vi "FPGA_GetRef.vi"() -> (0 "error out":errorcluster, 2 "FPGA_Ref":refnum<k20>)   [LabVIEW 2009]
uses:
  <vilib>/rvi/interface/nirviOpenFPGA/nirviOpenFPGA.xnode
  FPGA Bitfiles/scmproject.lvproj_FPGA Target_RobotFPGA.vi.lvbitx
  RobotFPGA.vi
  <vilib>/FPGAPlugInAG/cRIO-9074/nirviIntfOpen_cRIO-9074.vi
  <vilib>/userdefined/High Color/nirio_resource_hc.ctl
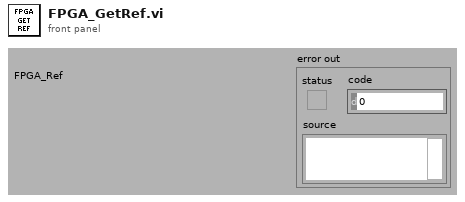
[diagram p1: front panel]
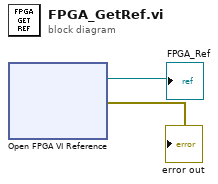
[diagram p0: block diagram]
diagram:
  n1 = xnode "Open FPGA VI Reference"() -> ("FPGA VI Reference Out"=→"FPGA_Ref":refnum<k20>, "error out"=→"error out":errorcluster)  [unwired: 2 in]
